vi "GetGraphRef.vi"(8 "error in (no error)":errorcluster, 11 "EpiWrapper in":refnum<class "EpiWrapper.lvclass">) -> (0 "error out":errorcluster, 2 "specific class reference":refnum<vi>, 3 "EpiWrapper out":refnum<class "EpiWrapper.lvclass">)   [LabVIEW 2012, in "EpiWrapper.lvclass"]
uses:
  EpiWrapper.lvclass
  EpiWrapper.lvclass/EpiWrapper.ctl
panel:
  out "XY Graph":cluster{"Y":dbl[], "Y":dbl[]}[](graph)
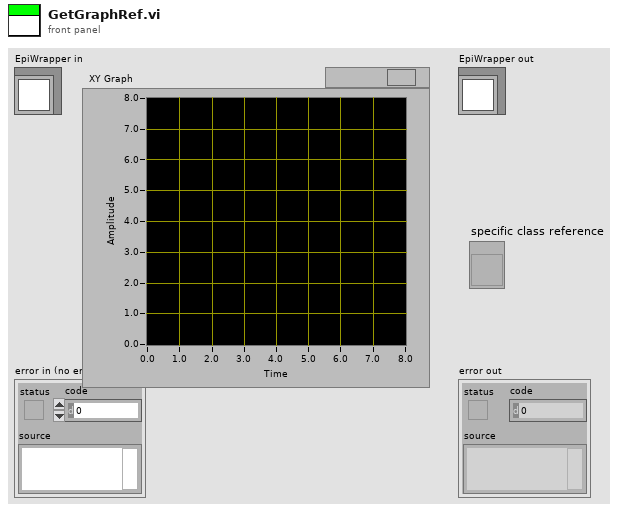
[diagram p1: front panel]
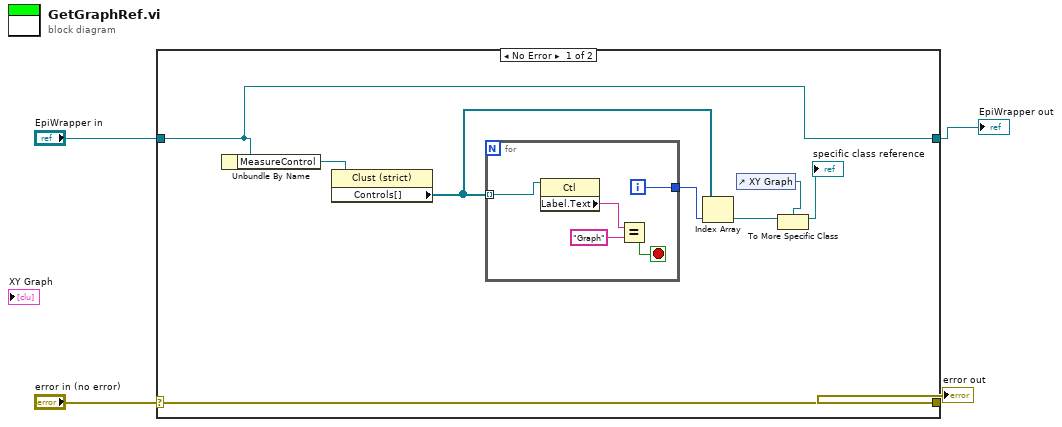
[diagram p0: block diagram]
diagram:
  n1 = case shown="No Error" "error in (no error)" {
    selector: "error in (no error)" -> [w12 w19]
    tunnel: [w12 w19] -> w3
    tunnel: [w5 w18] -> w1
    tunnel: "EpiWrapper in" -> [w5 w18]
    frame No Error {
      n2 = Unbundle By Name(w5) -> ("MeasureControl"=w11:refnum<vi>)
      n3 = property class="Clust (strict)"(reference=w11) -> ("Controls[]"=w9:refnum<vi>[])  [unwired: 1 in, 2 out]
      n4 = for {
        tunnel: w9 -> [w17] mode=indexing
        tunnel: [w13] -> w10
        i -> [w13]
        stop <- w14 stop-if-true
        n5 = property class="Ctl"(reference=w17) -> ("Label.Text"=w16:string)  [unwired: 1 in, 2 out]
        n6 = Equal?(x=w16, y="Graph") -> (x = y?=w14:bool)
      }
      n7 = Index Array(array=w9, index=w10) -> (element=w8:refnum<vi>)
      n8 = control-ref of="XY Graph"() -> (w7:refnum<vi>)
      n9 = To More Specific Class(target class=w7, reference=w8) -> (specific class reference=→"specific class reference":refnum<vi>)  [unwired: 1 in, 1 out]
    }
    frame Error {
    }
  }
  "error out" <- w3
  "EpiWrapper out" <- w1
